vi "TA_Generate_Filename.vi"(0 "Excitation Wavelength":string="800nm", 1 "Root Folder":path, 2 "Sample":string="sample", 3 "Solvent":string="solvent", 5 "Excitation Energy":string="1uj", 7 "Comments":string="XXXX", 9 "_scan/_average":enum16{"_scan", "_average"}(ring)=enum."_average", 11 "Current Scan":i16=1, 15 "Data Extension (.dat; .csv)":string=".dat") -> (12 "Folder":path, 13 "Filename":string, 14 "Filepath":path)   [LabVIEW 2025]
panel:
  out "error out":errorcluster
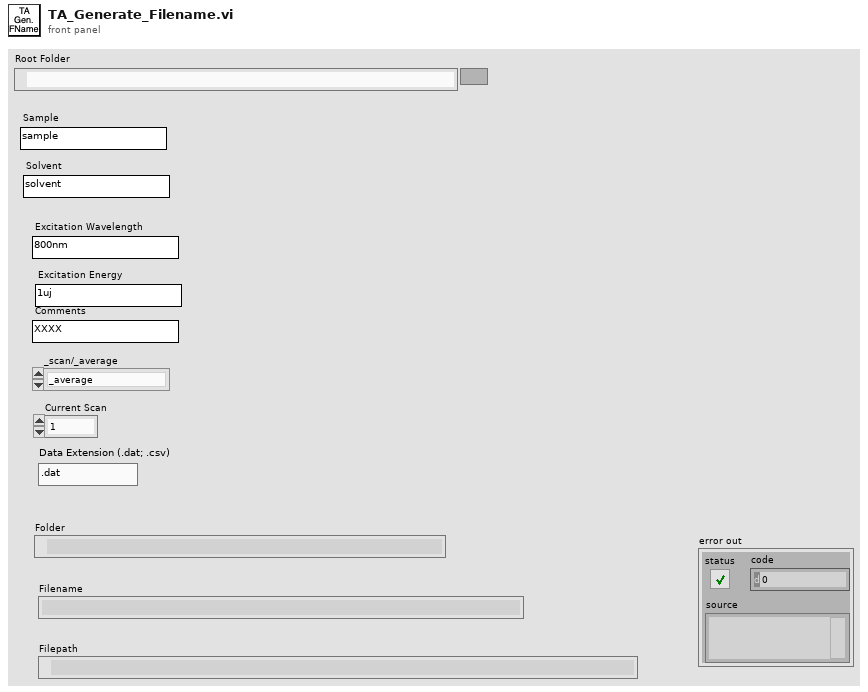
[diagram p1: front panel]
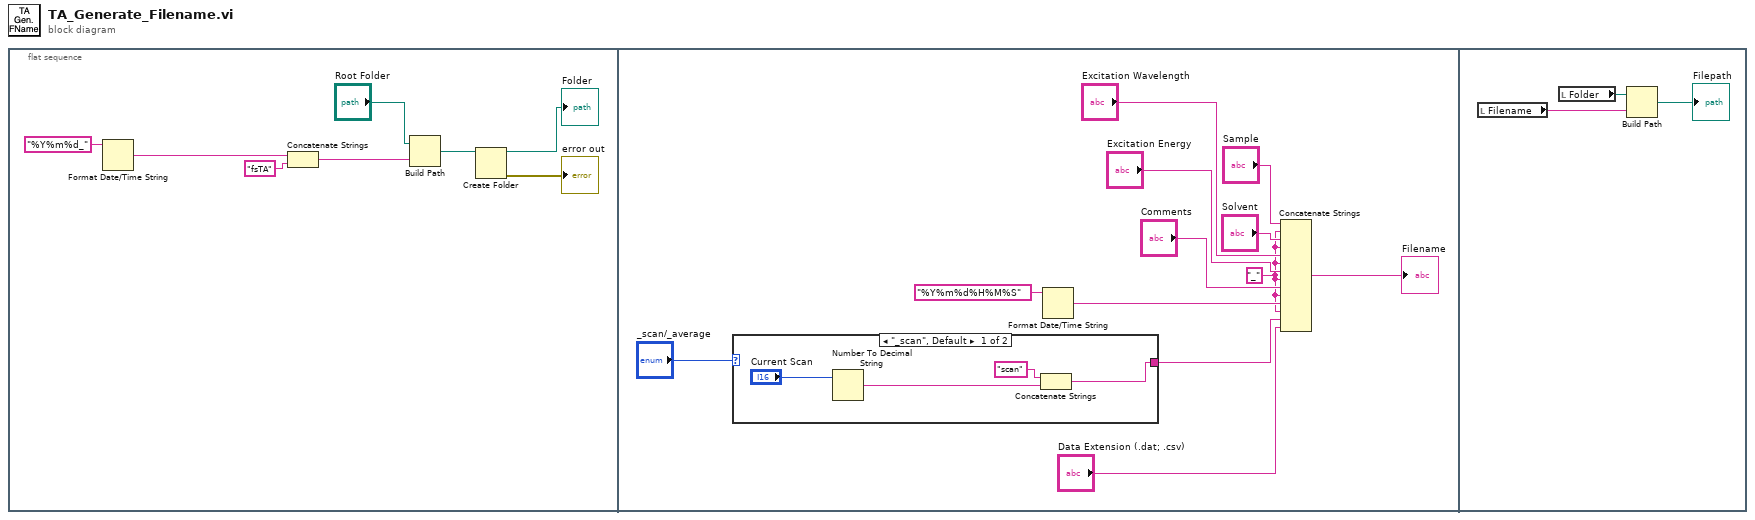
[diagram p0: block diagram]
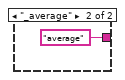
[diagram p2: hidden frame]
diagram:
  n1 = flat-sequence {
    frame #0 {
      n2 = Format Date/Time String(time format string (%c)="%Y%m%d_") -> (date/time string=w5:string)  [unwired: 2 in]
      n3 = Concatenate Strings "Concatenate Strings"(w5, "fsTA" ("String")) -> (w4:string)
      n4 = Build Path(base path="Root Folder", name or relative path=w4) -> (appended path=w8:path)
      n5 = Create Folder(path (use dialog)=w8) -> (created path=→"Folder":path, error out=→"error out":errorcluster)  [unwired: 2 in, 1 out]
    }
    frame #1 {
      w10 = "_" ("string")
      n6 = case shown="\"_scan\", Default" "_scan/_average" {
        tunnel: [w22 "average"] -> w11
        frame "_scan", Default {
          n7 = Number To Decimal String(number="Current Scan") -> (decimal integer string=w23:string)  [unwired: 1 in]
          n8 = Concatenate Strings("scan" ("string"), w23) -> (w22:string)
        }
        frame "_average" {
        }
      }
      n9 = Format Date/Time String(time format string (%c)="%Y%m%d%H%M%S") -> (date/time string=w15:string)  [unwired: 2 in]
      n10 = Concatenate Strings "Concatenate Strings"("Sample", w10, "Solvent", w10, "Excitation Wavelength", w10, "Excitation Energy", w10, "Comments", w10, w15, w10, w11, "Data Extension (.dat; .csv)") -> (→"Filename":string)
    }
    frame #2 {
      n11 = local read "Filename"() -> (w27:string)
      n12 = local read "Folder"() -> (w28:path)
      n13 = Build Path(base path=w28, name or relative path=w27) -> (appended path=→"Filepath":path)
    }
  }
